vi "CalculateAllAverages.vi"(10 "Instrument":string, 11 "Path To TRF Folder":path) -> (0 "Complex Average":cdb[](array[numeric]), 1 "FRF Spectra":cluster{dbl, "df":dbl, "FFT {X}":dbl[]}[](graph), 3 "Array":path[](array[path]))   [LabVIEW 2022 SP3]
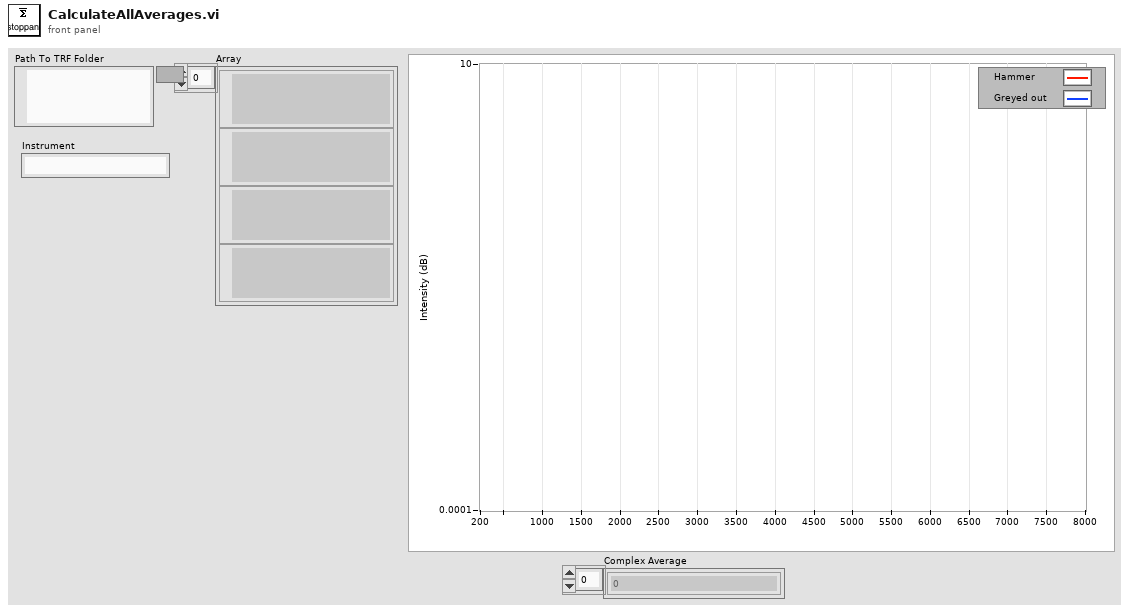
[diagram p1: front panel]
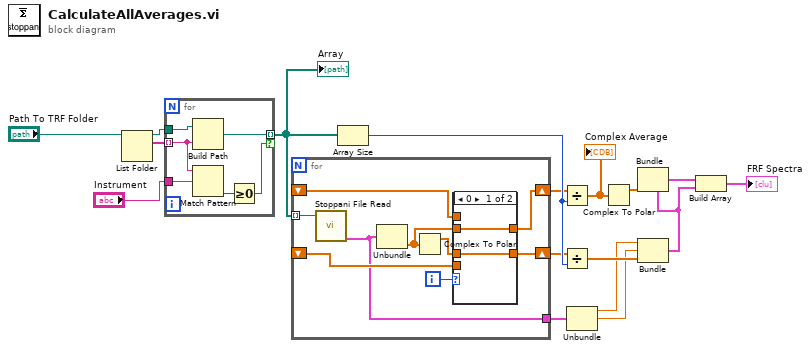
[diagram p0: block diagram]
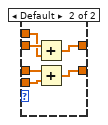
[diagram p2: hidden frame]
diagram:
  n1 = List Folder(path="Path To TRF Folder") -> (path out=w10:path, filenames=w9:string[])  [unwired: 3 in, 2 out]
  n2 = for {
    tunnel: w9 -> [w21] mode=indexing
    tunnel: "Instrument" -> [w23]
    tunnel: w10 -> [w20]
    tunnel: [w18] -> w15 mode=indexing if=w19
    n3 = Build Path(base path=w20, name or relative path=w21) -> (appended path=w18:path)
    n4 = Match Pattern(string=w21, regular expression=w23) -> (offset past match=w22:i32)  [unwired: 1 in, 3 out]
    n5 = Greater Or Equal To 0?(x=w22) -> (x >= 0?=w19:bool)
  }
  "Array" <- w15
  n6 = for {
    tunnel: w15 -> [w32] mode=indexing
    shift-right: [w30] -> w14
    shift-left: _ -> [w29]
    shift-right: [w27] -> w12
    shift-left: _ -> [w26]
    tunnel: [w24] -> w4
    i -> [w25]
    n7 = call "Stoppani File Read.vi"("String in"=w32) -> ("Complex FRF"=w24:cluster{"t0":dbl, "dt":dbl, "Y":cdb[]})  [unwired: 2 in, 3 out]
    n8 = Unbundle(w24) -> ("Y"=w28:cdb[])  [unwired: 2 out]
    n9 = Complex To Polar(r * e^(i*theta)=w28) -> (r=w31:dbl[])  [unwired: 1 out]
    n10 = case shown="0" w25 {
      tunnel: w31 -> [w34 w40]
      tunnel: [w34 w39] -> w30
      tunnel: w29 -> [_ w38]
      tunnel: w28 -> [w33 w37]
      tunnel: [w33 w36] -> w27
      tunnel: w26 -> [_ w35]
      frame 0 {
      }
      frame Default {
        n11 = Add(x=w37, y=w35) -> (x+y=w36:cdb[])
        n12 = Add(x=w40, y=w38) -> (x+y=w39:dbl[])
      }
    }
  }
  n13 = Array Size(array=w15) -> (size(s)=w16:i32)
  n14 = Divide(x=w12, y=w16) -> (x/y=w13:cdb[])
  "Complex Average" <- w13
  n15 = Divide(x=w14, y=w16) -> (x/y=w8:dbl[])
  n16 = Unbundle(w4) -> ("t0"=w3:dbl, "dt"=w2:dbl)  [unwired: 1 out]
  n17 = Complex To Polar(r * e^(i*theta)=w13) -> (r=w6:dbl[])  [unwired: 1 out]
  n18 = Bundle("t0"=w3, "dt"=w2, w8) -> (w1:cluster{"t0":dbl, "dt":dbl, dbl[]})  [unwired: 1 in]
  n19 = Bundle(cluster=w1, w6) -> (w7:cluster{"t0":dbl, "dt":dbl, dbl[]})  [unwired: 2 in]
  n20 = Build Array(w7, w1) -> (→"FRF Spectra":cluster{"t0":dbl, "dt":dbl, dbl[]}[])
